vi "setUp.vi"(8 "error in":errorcluster, 11 "reference in":refnum<class "Scripting.lvclass">) -> (0 "error out":errorcluster, 3 "reference out":refnum<class "Scripting.lvclass">)   [LabVIEW 2020, in "Scripting.lvclass"]
doc: "setUp runs prior to the test method during test execution. Use this method to initialize any object data required by your tests."
uses:
  Scripting.lvclass
  C:/Program Files (x86)/National Instruments/LabVIEW 2020/vi.lib/addons/_JKI Toolkits/VI Tester/TestCase.llb/TestCase.lvclass
  Scripting.lvclass/Scripting.ctl
  <vilib>/addons/_JKI Toolkits/VI Tester/TestCase.llb/TestCase.lvclass
  niveristand-custom-device-testing-tools/VeriStandTestUtilities/VeriStandTestUtilities.lvlib
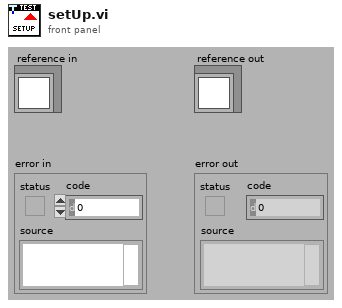
[diagram p1: front panel]
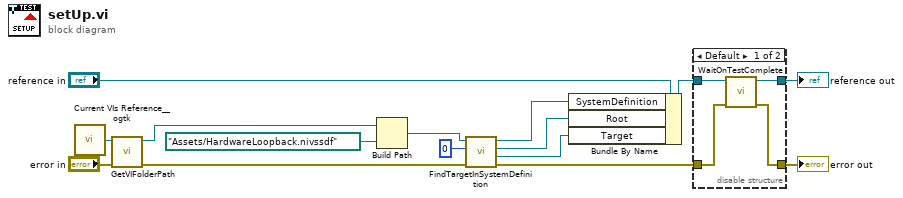
[diagram p0: block diagram]
diagram:
  n1 = call <userlib>:"Current VIs Reference__ogtk.vi"() -> ("Current VI's reference"=w13:refnum<vi>)  [unwired: 5 in]
  n2 = call "GetVIFolderPath.vi"("error in (no error)"="error in", "VI Reference in"=w13) -> ("error out"=w2:errorcluster, "VI Folder Path out"=w12:path)  [unwired: 8 in]
  n3 = Build Path(base path=w12, name or relative path=path "Assets/HardwareLoopback.nivssdf" ("Absolute or Relative Path")) -> (appended path=w7:path)
  n4 = call "FindTargetInSystemDefinition.vi"("error in"=w2, "target index"=0 ("index"), "system definition path"=w7) -> ("error out"=w1:errorcluster, "Target"=w3:refnum<k24>, "Root"=w4:refnum<k24>, "System Definition"=w5:refnum<k24>)  [unwired: 5 in]
  n5 = Bundle By Name(cluster="reference in", "SystemDefinition"=w5, "Root"=w4, "Target"=w3) -> (w8:refnum<class "Scripting.lvclass">)
  n6 = disable-structure shown="Default" {
    disable-tunnel: w1 -> [w19 w20]
    disable-tunnel: [w18 w20] -> w15
    disable-tunnel: [w17 w21] -> w14
    disable-tunnel: w8 -> [w16 w21]
    frame condition #0 (active) {
      n7 = call <vilib>:"WaitOnTestComplete.vi"("error in (no error)"=w19, "TestCase in"=w16) -> ("error out"=w18:errorcluster, "TestCase out"=w17:refnum<class "Scripting.lvclass">)  [unwired: 8 in]
    }
    frame condition #1 {
    }
  }
  "error out" <- w15
  "reference out" <- w14
